vi "SwerveCornerKinematics.vi"(9 "J2X":dbl, 11 "Pivot Module":i32) -> (0 "Magnitude 3":dbl, 1 "Magnitude 2":dbl, 2 "Magnitude 1":dbl, 3 "Magnitude 0":dbl, 4 "Wheel Angle 2":dbl, 5 "Wheel Angle 1":dbl, 6 "Wheel Angle 3":dbl, 7 "Wheel Angle 0":dbl)   [LabVIEW 2019]
doc: "Performs the kinematics for a square four wheel swerve robot with a center of rotation at the one of the four corners of the robot. Swerve module #0 is located in the front right corner and the modules increment in the counter-clockwise direction."
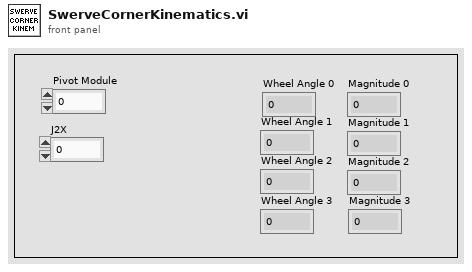
[diagram p1: front panel]
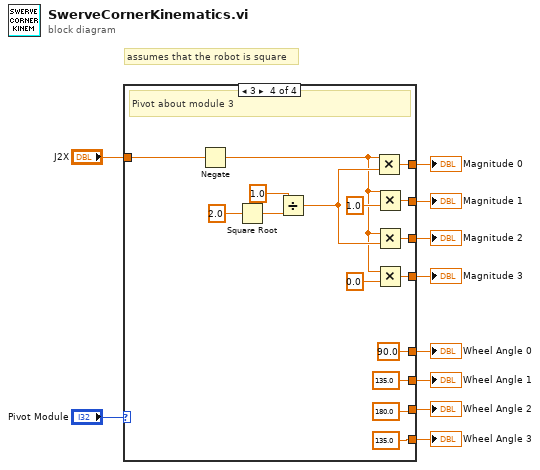
[diagram p0: block diagram]
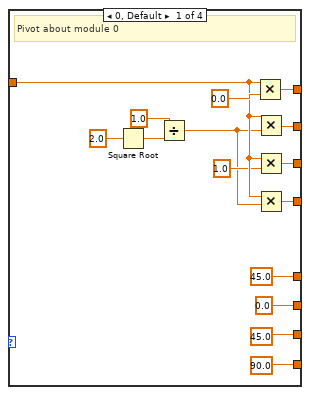
[diagram p2: hidden frame]
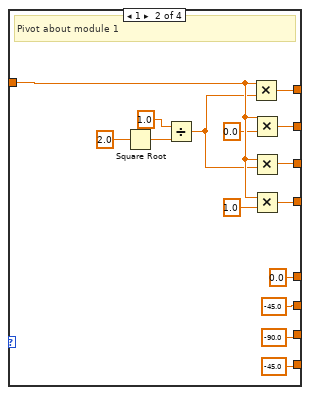
[diagram p3: hidden frame]
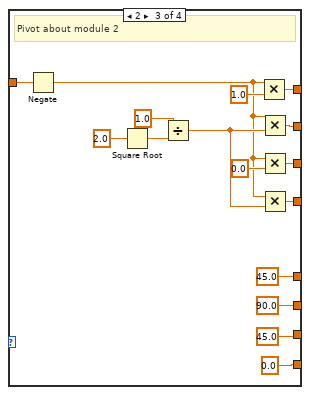
[diagram p4: hidden frame]
diagram:
  # "assumes that the robot is square"
  n1 = case shown="3" "Pivot Module" {
    tunnel: [45.0 0.0 45.0 90.0] -> w9
    tunnel: [0.0 -45.0 90.0 135.0] -> w8
    tunnel: [45.0 -90.0 45.0 180.0] -> w7
    tunnel: [90.0 -45.0 0.0 135.0] -> w6
    tunnel: "J2X" -> [w20 w37 w53 w69]
    tunnel: [w25 w32 w48 w68] -> w5
    tunnel: [w23 w31 w47 w67] -> w4
    tunnel: [w22 w30 w46 w66] -> w3
    tunnel: [w21 w29 w45 w65] -> w2
    frame 0, Default {
      # "Pivot about module 0"
      n2 = Square Root(x=2.0) -> (sqrt(x)=w17:dbl)
      n3 = Divide(x=1.0, y=w17) -> (x/y=w15:dbl)
      n4 = Multiply(x=w20, y=0.0) -> (x*y=w25:dbl)
      n5 = Multiply(x=w20, y=w15) -> (x*y=w23:dbl)
      n6 = Multiply(x=w20, y=1.0) -> (x*y=w22:dbl)
      n7 = Multiply(x=w20, y=w15) -> (x*y=w21:dbl)
    }
    frame 1 {
      # "Pivot about module 1"
      n8 = Square Root(x=2.0) -> (sqrt(x)=w40:dbl)
      n9 = Divide(x=1.0, y=w40) -> (x/y=w26:dbl)
      n10 = Multiply(x=w37, y=w26) -> (x*y=w32:dbl)
      n11 = Multiply(x=w37, y=0.0) -> (x*y=w31:dbl)
      n12 = Multiply(x=w37, y=w26) -> (x*y=w30:dbl)
      n13 = Multiply(x=w37, y=1.0) -> (x*y=w29:dbl)
    }
    frame 2 {
      # "Pivot about module 2"
      n14 = Negate(x=w53) -> (-x=w41:dbl)
      n15 = Square Root(x=2.0) -> (sqrt(x)=w55:dbl)
      n16 = Divide(x=1.0, y=w55) -> (x/y=w42:dbl)
      n17 = Multiply(x=w41, y=1.0) -> (x*y=w48:dbl)
      n18 = Multiply(x=w41, y=w42) -> (x*y=w47:dbl)
      n19 = Multiply(x=w41, y=0.0) -> (x*y=w46:dbl)
      n20 = Multiply(x=w41, y=w42) -> (x*y=w45:dbl)
    }
    frame 3 {
      # "Pivot about module 3"
      n21 = Negate(x=w69) -> (-x=w57:dbl)
      n22 = Square Root(x=2.0) -> (sqrt(x)=w71:dbl)
      n23 = Divide(x=1.0, y=w71) -> (x/y=w58:dbl)
      n24 = Multiply(x=w57, y=w58) -> (x*y=w68:dbl)
      n25 = Multiply(x=w57, y=1.0) -> (x*y=w67:dbl)
      n26 = Multiply(x=w57, y=w58) -> (x*y=w66:dbl)
      n27 = Multiply(x=w57, y=0.0) -> (x*y=w65:dbl)
    }
  }
  "Wheel Angle 0" <- w9
  "Wheel Angle 1" <- w8
  "Wheel Angle 2" <- w7
  "Wheel Angle 3" <- w6
  "Magnitude 0" <- w5
  "Magnitude 1" <- w4
  "Magnitude 2" <- w3
  "Magnitude 3" <- w2
